vi "KM_Readout.vi"() -> ()   [LabVIEW 2015]
uses:
  <instrlib>/Zurich Instruments LabOne/Public/Data/ziTypePollType.ctl
  ZI_Frontpanel.ctl
  HF_FrontPanel.ctl
  <vilib>/Analysis/baseanly.llb/Mean (DBL).vi
  MQM Data Transfer_KM.vi
  <instrlib>/Zurich Instruments LabOne/Public/Data/ziGetEventAuxInSample.vi
  <instrlib>/Zurich Instruments LabOne/Public/Data/ziGetEventDemodSample.vi
  <instrlib>/Zurich Instruments LabOne/Zurich Instruments LabOne.lvlib
  <vilib>/Analysis/NI_AALBase.lvlib
panel:
  out "AUX Input 5":dbl[](graph)
  out "ziValueType 5":T1
  in  "stop 2":bool
  out "ZI HFLI":T2 {"Lockin 1 Demod 0"."R(V)" format="%#_6p"}
  out "ZI MFLI":T3 {"Lockin 1 Demod 3"."R(V)" format="%#_6p"; "Lockin 1 Demod 2"."R(V)" format="%#_6p"; "Lockin 4 Demod 1"."R(V)" format="%#_6p"; "Lockin 3 Demod 1"."R(V)" format="%#_6p"; "Lockin 2 Demod 1"."R(V)" format="%#_6p"; "Lockin 1 Demod 1"."R(V)" format="%#_6p"; "Lockin 4 Demod 0"."R(V)" format="%#_6p"; "Lockin 3 Demod 0"."R(V)" format="%#_6p"; "Lockin 2 Demod 0"."R(V)" format="%#_6p"; "Lockin 1 Demod 0"."R(V)" format="%#_6p"}
  out "AUX Input 4":dbl[](graph)
  out "ziValueType 4":T1
  out "AUX Input 3":dbl[](graph)
  out "ziValueType 3":T1
  out "AUX Input 2":dbl[](graph)
  out "ziValueType 2":T1
  in  "stop":bool
  out "ziValueType":T1
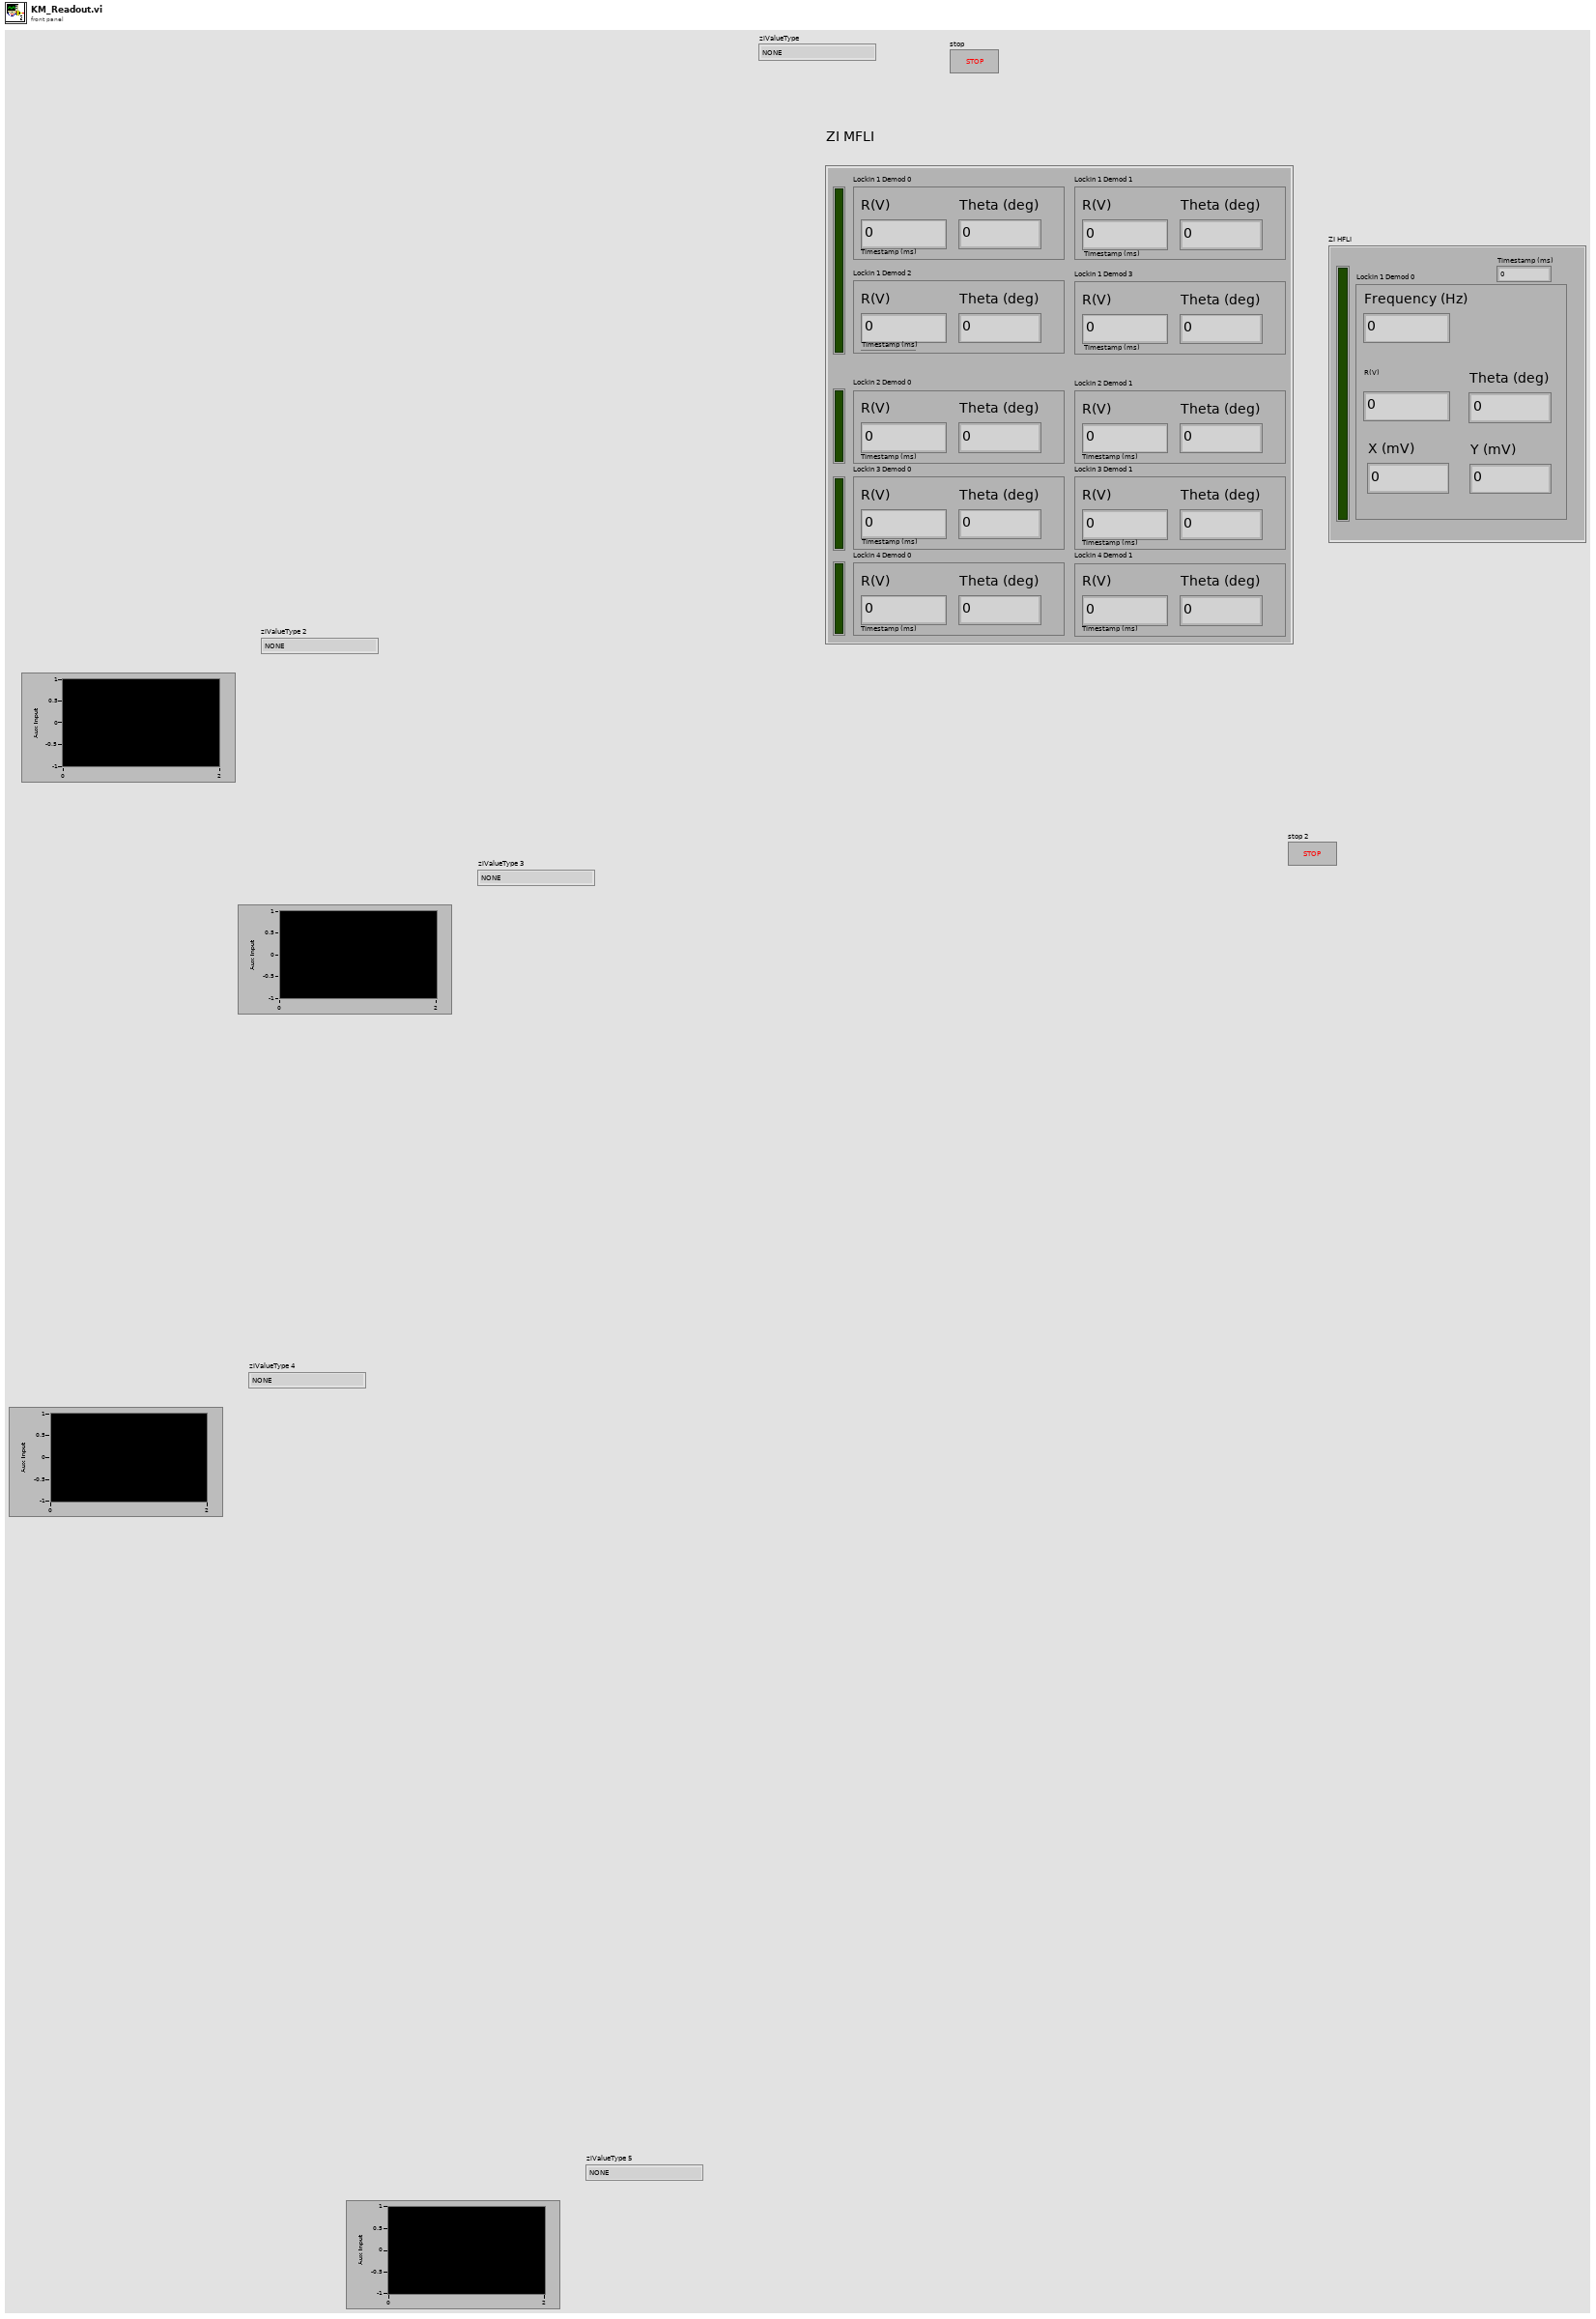
[diagram p1: front panel]
types:
  T1 = typedef "Zurich Instruments LabOne.lvlib/ziTypePollType.ctl" = enum16{"NONE", "DOUBLE_DATA", "INTEGER_DATA", "DEMOD_SAMPLE", "SCOPE_WAVE_HF2", "AUXIN_SAMPLE", "DIO_SAMPLE", "BYTE_ARRAY", "PWA_WAVE", "9", "10", "11", "12", "13", "14", "15", "TREE_CHANGE_DEPRI", "17", "ERROR", "19", "20", "21", "22", "23", "24", "25", "26", "27", "28", "29", "30", "31", "DOUBLE_DATA_TS", "INTEGER_DATA_TS", "34", "SCOPE_WAVE", "36", "37", "BYTE_ARRAY_TS", "39", "40", "41", "42", "43", "44", "45", "CNT_DATA", "47", "TREE_CHANGE", "49", "50", "51", "52", "53", "54", "55", "56", "57", "58", "59", "60", "61", "62", "63", "SWEEPER_DATA", "SPECTRUM_DATA", "ADVISOR_DATA", "67", "IMP_DATA"}
  T2 = typedef "HF_FrontPanel.ctl" = cluster{"Lockin 1 Demod 0":cluster{"R(V)":dbl, "Theta (deg)":dbl, "Frequency (Hz)":dbl, "X (mV)":dbl, "Y (mV)":dbl}, "LI1 active":bool, "Timestamp (ms)":u32}
  T3 = typedef "ZI_Frontpanel.ctl" = cluster{"Lockin 1 Demod 0":cluster{"R(V)":dbl, "Theta (deg)":dbl, "Timestamp (ms)":u32}, "Lockin 2 Demod 0":cluster{"R(V)":dbl, "Theta (deg)":dbl, "Timestamp (ms)":u32}, "Lockin 3 Demod 0":cluster{"R(V)":dbl, "Theta (deg)":dbl, "Timestamp (ms)":u32}, "Lockin 4 Demod 0":cluster{"R(V)":dbl, "Theta (deg)":dbl, "Timestamp (ms)":u32}, "Lockin 1 Demod 1":cluster{"R(V)":dbl, "Theta (deg)":dbl, "Timestamp (ms)":u32}, "Lockin 2 Demod 1":cluster{"R(V)":dbl, "Theta (deg)":dbl, "Timestamp (ms)":u32}, "Lockin 3 Demod 1":cluster{"R(V)":dbl, "Theta (deg)":dbl, "Timestamp (ms)":u32}, "Lockin 4 Demod 1":cluster{"R(V)":dbl, "Theta (deg)":dbl, "Timestamp (ms)":u32}, "Lockin 1 Demod 2":cluster{"R(V)":dbl, "Theta (deg)":dbl, "Timestamp (ms)":u32}, "Lockin 1 Demod 3":cluster{"R(V)":dbl, "Theta (deg)":dbl, "Timestamp (ms)":u32}, "LI1 active":bool, "LI2 active":bool, "LI3 active":bool, "LI4 active":bool}
  T4 = cluster{"ZI IP List[0]":string, "ZI IP List[1]":string, "ZI IP List[2]":string, "ZI IP List[3]":string, "ZI IP List[4]":string, "ZI IP List[5]":string, "ZI IP List[6]":string, "ZI IP List[7]":string, "ZI IP List[8]":string}
  T5 = typedef "Zurich Instruments LabOne.lvlib/ziTypeHandle.ctl" = cluster{"handleValid":bool, "Conn":u64, "Path Prefix":string, "Handle":u64, "Connected":bool, "Clockbase(s)":dbl}
  T6 = typedef "Zurich Instruments LabOne.lvlib/ziTypeAuxInSample.ctl" = cluster{"Timestamp (ticks)":u64[], "Val Ch0 (V)":dbl[], "Val Ch1 (V)":dbl[]}
  T7 = typedef "ziTypeDemodSampleEx.ctl" = cluster{"Timestamps (ticks)":u64[], "X (Vrms)":dbl[], "Y (Vrms)":dbl[], "Osc Phase (rad)":dbl[], "Freq (Hz)":dbl[], "DIO":u32[], "Aux In 0 (V)":dbl[], "Aux In 1 (V)":dbl[], "Trigger":u32[]}
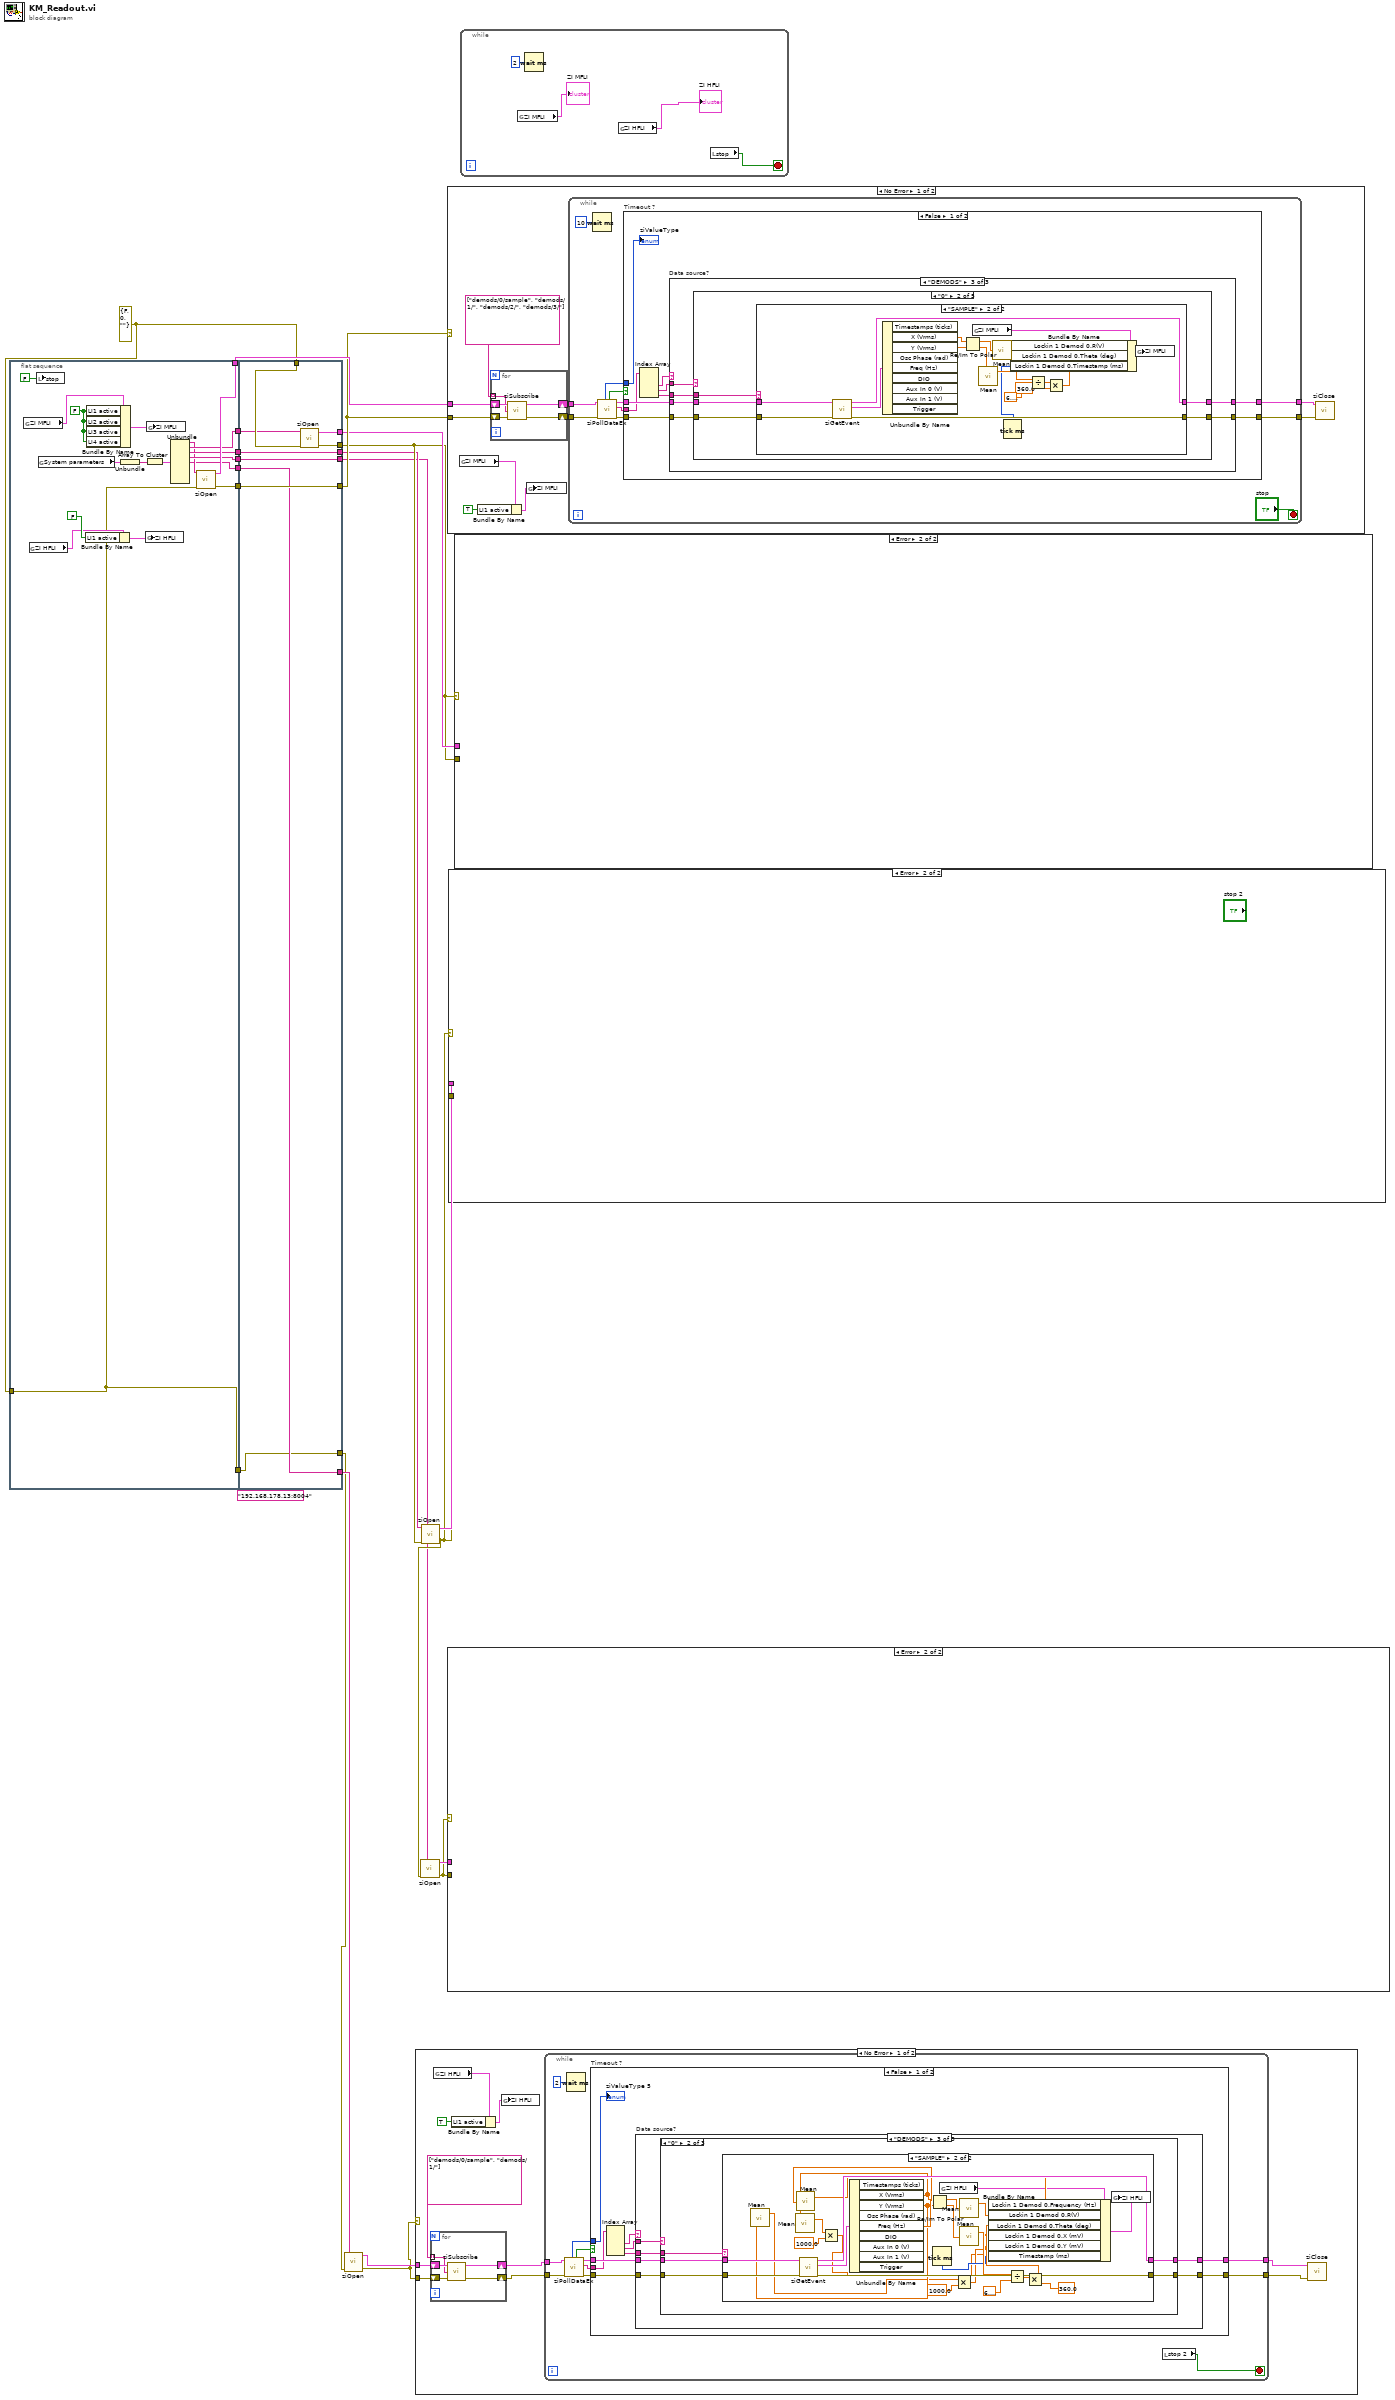
[diagram p0: block diagram]
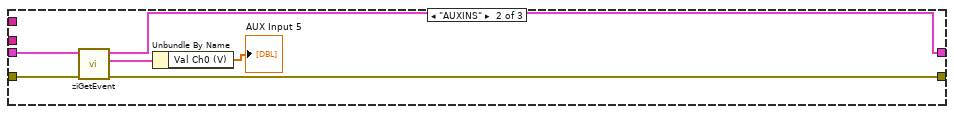
[diagram p3: hidden frame]
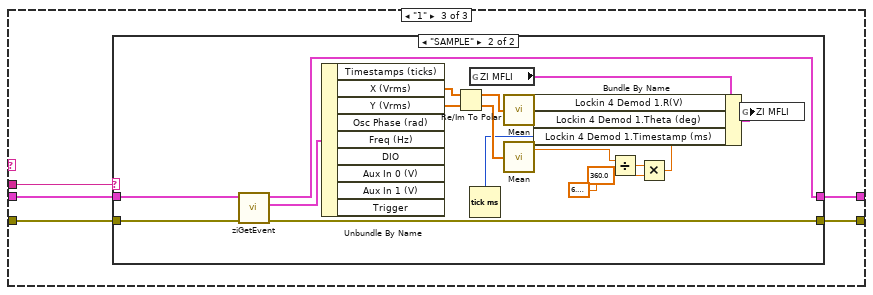
[diagram p6: hidden frame]
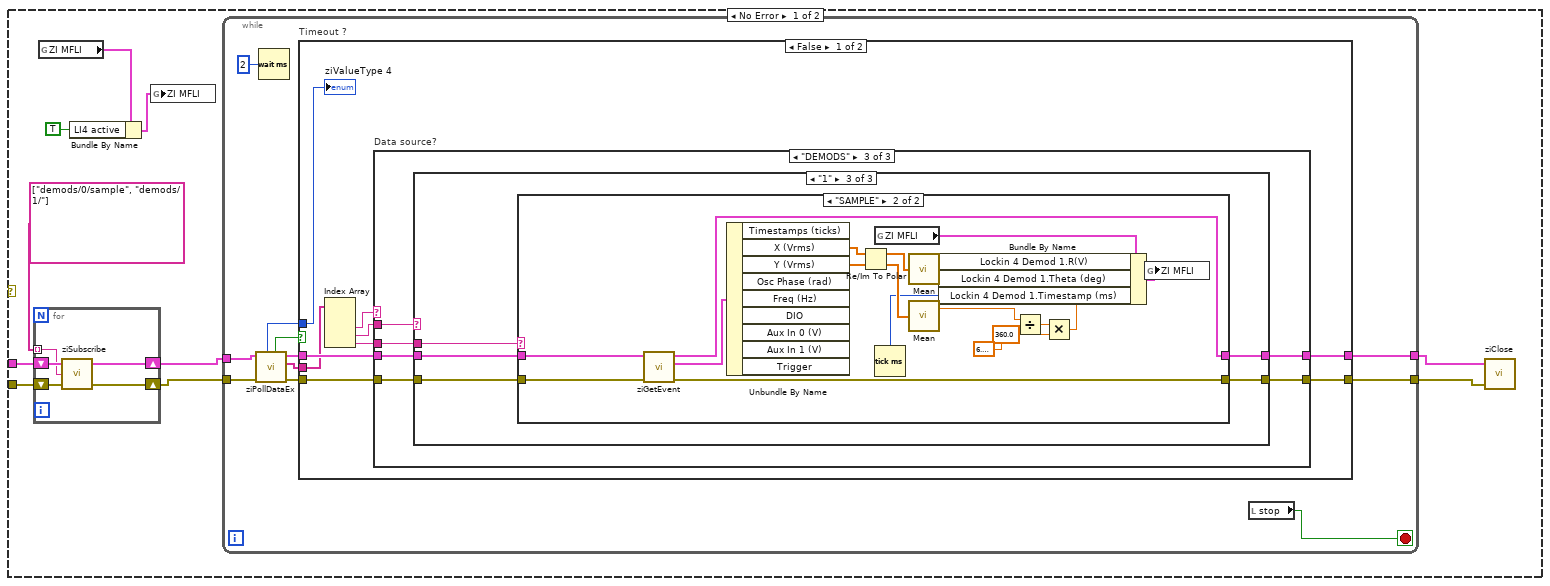
[diagram p10: hidden frame]
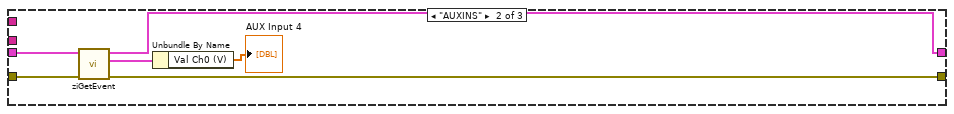
[diagram p12: hidden frame]
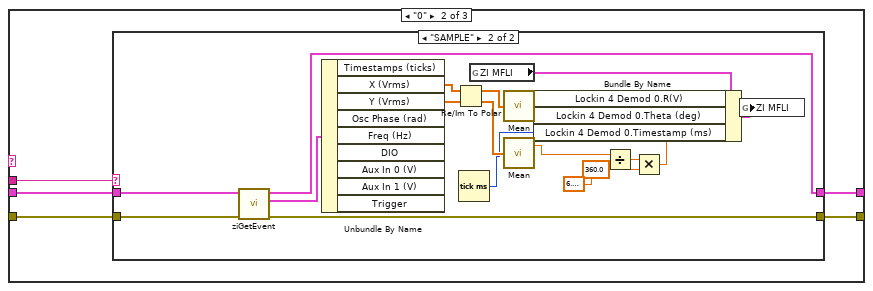
[diagram p14: hidden frame]
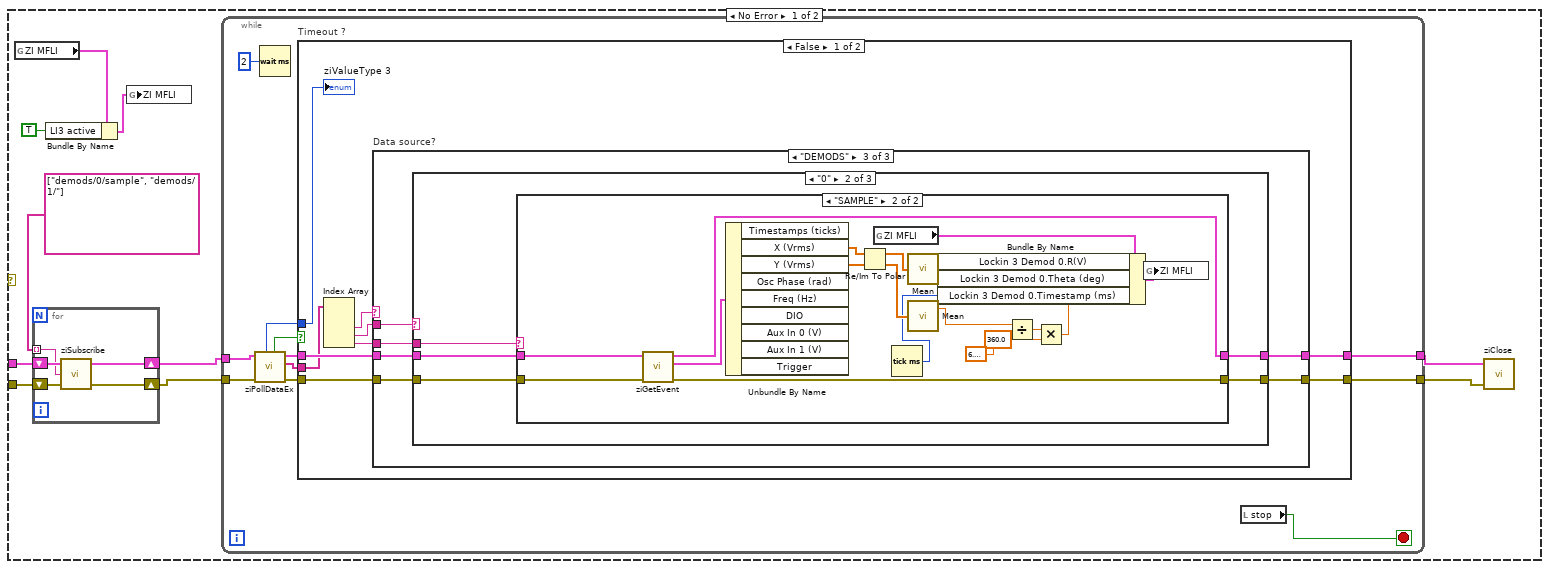
[diagram p18: hidden frame]
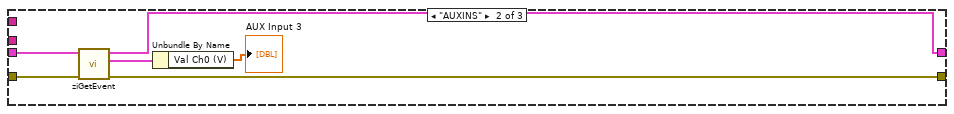
[diagram p20: hidden frame]
diagram:
  (unwired) "192.168.178.13:8004"
  w15 = errorcluster {"status"=FALSE, "code"=0, "source"=""} ("Error In")
  n1 = flat-sequence {
    tunnel: [w38] -> w19
    tunnel: [w37] -> w17
    tunnel: w15 -> [w22]
    tunnel: [w31] -> w12
    tunnel: [w30] -> w11
    tunnel: [w29] -> w10
    tunnel: [w23] -> w6
    tunnel: [w22] -> w2
    tunnel: [w48] -> w18
    tunnel: w17 -> [w48]
    tunnel: w15 -> [w47]
    tunnel: [w46] -> w14
    tunnel: [w45] -> w16
    tunnel: w12 -> [w44]
    tunnel: [w43] -> w9
    tunnel: w11 -> [w43]
    tunnel: [w42] -> w5
    tunnel: w10 -> [w42]
    tunnel: w6 -> [w41]
    tunnel: [w41] -> w4
    tunnel: w2 -> [w40]
    tunnel: [w40] -> w1
    frame #0 {
      w35 = FALSE ("LI1 active")
      n2 = global read "MQM Data Transfer_KM.vi" "ZI MFLI"() -> (w28:T3)
      n3 = global read "MQM Data Transfer_KM.vi" "ZI HFLI"() -> (w26:T2)
      n4 = local write "stop"(FALSE ("stop")) -> ()
      n5 = global read "MQM Data Transfer_KM.vi" "System parameters"() -> (w34:cluster{"ZI IP List":string[]})
      n6 = Bundle By Name(cluster=w26, "LI1 active"=FALSE) -> (w25:T2)
      n7 = Bundle By Name(cluster=w28, "LI1 active"=w35, "LI2 active"=w35, "LI3 active"=w35, "LI4 active"=w35) -> (w36:T3)
      n8 = Unbundle(w34) -> ("ZI IP List"=w33:string[])
      n9 = Array To Cluster(array=w33) -> (cluster=w32:T4)
      n10 = global write "MQM Data Transfer_KM.vi" "ZI HFLI"(w25) -> ()
      n11 = global write "MQM Data Transfer_KM.vi" "ZI MFLI"(w36) -> ()
      n12 = Unbundle(w32) -> ("ZI IP List[0]"=w24:string, "ZI IP List[1]"=w31:string, "ZI IP List[2]"=w30:string, "ZI IP List[3]"=w29:string, "ZI IP List[4]"=w23:string)  [unwired: 4 out]
      n13 = call <instrlib>:"ziOpen.vi"("Error In"=w22, "Address"=w24) -> ("Error Out"=w37:errorcluster, "HandleOut"=w38:T5)  [unwired: 3 out]
    }
    frame #1 {
      n14 = call <instrlib>:"ziOpen.vi"("Error In"=w47, "Address"=w44) -> ("Error Out"=w46:errorcluster, "HandleOut"=w45:T5)  [unwired: 3 out]
    }
  }
  n15 = call <instrlib>:"ziOpen.vi"("Error In"=w1, "Address"=w4) -> ("Error Out"=w7:errorcluster, "HandleOut"=w8:T5)  [unwired: 3 out]
  n16 = case shown="No Error" w7 {
    tunnel: w8 -> [w58 _]
    tunnel: w7 -> [w57 _]
    frame No Error {
      n17 = for {
        shift-right: [w63] -> w55
        shift-left: w58 -> [w61]
        shift-right: [w62] -> w54
        shift-left: w57 -> [w60]
        tunnel: string[] ["demods/0/sample", "demods/1/"] -> [w59] mode=indexing
        n18 = call <instrlib>:"ziSubscribe.vi"("error in"=w60, "Path ()"=w59, "Handle In"=w61) -> ("error out"=w62:errorcluster, "Handle Out"=w63:T5)  [unwired: 1 in]
      }
      n19 = global read "MQM Data Transfer_KM.vi" "ZI HFLI"() -> (w51:T2)
      n20 = Bundle By Name(cluster=w51, "LI1 active"=TRUE) -> (w49:T2)
      n21 = global write "MQM Data Transfer_KM.vi" "ZI HFLI"(w49) -> ()
      n22 = while {
        tunnel: w55 -> [w69]
        tunnel: w54 -> [w68]
        tunnel: [w67] -> w52
        tunnel: [w66] -> w53
        stop <- w65 stop-if-true
        n23 = call <instrlib>:"ziPollDataEx.vi"("error in"=w68, "Handle In"=w69) -> ("error out"=w72:errorcluster, "PathArray"=w70:string[], "Handle Out"=w74:T5, "Timed Out"=w73:bool, "ziValueType"=w71:T1)  [unwired: 2 in, 3 out]
        n24 = Wait (ms)(milliseconds to wait=u32 2) -> ()  [unwired: 1 out]
        n25 = case "Timeout ?" shown="False" w73 {
          tunnel: w74 -> [w83 w159]
          tunnel: [w82 w159] -> w66
          tunnel: w72 -> [w81 w158]
          tunnel: [w80 w158] -> w67
          tunnel: w71 -> [w79 _]
          tunnel: w70 -> [w78 _]
          frame False {
            n26 = Index Array(array=w78) -> (element #2=w75:string, element #3=w76:string, element #4=w77:string)  [unwired: 4 in, 1 out]
            n27 = case "Data source?" shown="\"DEMODS\"" w75 {
              tunnel: w83 -> [w85 w91 w97]
              tunnel: [w85 w89 w96] -> w82
              tunnel: w81 -> [w84 w88 w95]
              tunnel: [w84 w87 w94] -> w80
              tunnel: w76 -> [_ _ w93]
              tunnel: w77 -> [_ _ w92]
              frame Default {
              }
              frame "AUXINS" {
                n28 = call-poly <instrlib>:"ziGetEvent.vi"("Error In"=w88, "Handle In"=w91) -> ("Error Out"=w87:errorcluster, "AuxIn Out"=w90:T6, "Handle Out"=w89:T5)  [unwired: 7 in]
                n29 = Unbundle By Name(w90) -> ("Val Ch0 (V)"=→"AUX Input 5":dbl[])
              }
              frame "DEMODS" {
                n30 = case shown="\"0\"" w93 {
                  tunnel: w97 -> [w99 w104 w137]
                  tunnel: [w99 w103 w136] -> w96
                  tunnel: w95 -> [w98 w102 w135]
                  tunnel: [w98 w101 w134] -> w94
                  tunnel: w92 -> [_ w100 w133]
                  frame Default {
                  }
                  frame "0" {
                    n31 = case shown="\"SAMPLE\"" w100 {
                      tunnel: w104 -> [w106 w132]
                      tunnel: [w106 w130] -> w103
                      tunnel: w102 -> [w105 w129]
                      tunnel: [w105 w128] -> w101
                      frame Default {
                      }
                      frame "SAMPLE" {
                        n32 = call-poly <instrlib>:"ziGetEvent.vi"("Error In"=w129, "Handle In"=w132) -> ("Error Out"=w128:errorcluster, "Demod Sample Out"=w131:T7, "Handle Out"=w130:T5)  [unwired: 7 in]
                        n33 = Unbundle By Name(w131) -> ("X (Vrms)"=w116:dbl[], "Y (Vrms)"=w115:dbl[], "Freq (Hz)"=w118:dbl[])  [unwired: 6 out]
                        n34 = call-poly <vilib>:"Mean.vi"("X"=w115) -> ("mean"=w111:dbl)  [unwired: 1 out]
                        n35 = call-poly <vilib>:"Mean.vi"("X"=w116) -> ("mean"=w108:dbl)  [unwired: 1 out]
                        n36 = call-poly <vilib>:"Mean.vi"("X"=w118) -> ("mean"=w117:dbl)  [unwired: 1 out]
                        n37 = Multiply(x=w108, y=1000.0) -> (x*y=w107:dbl)
                        n38 = Re/Im To Polar(2:w115, 3:w116) -> (0:w126:dbl[], 1:w127:dbl[])
                        n39 = Tick Count (ms)() -> (millisecond timer value=w119:u32)
                        n40 = global read "MQM Data Transfer_KM.vi" "ZI HFLI"() -> (w114:T2)
                        n41 = Multiply(x=w111, y=1000.0) -> (x*y=w110:dbl)
                        n42 = call-poly <vilib>:"Mean.vi"("X"=w127) -> ("mean"=w122:dbl)  [unwired: 1 out]
                        n43 = call-poly <vilib>:"Mean.vi"("X"=w126) -> ("mean"=w121:dbl)  [unwired: 1 out]
                        n44 = Divide(x=w121, y=6.283185307179586) -> (x/y=w124:dbl)
                        n45 = Multiply(x=w124, y=360.0) -> (x*y=w120:dbl)
                        n46 = Bundle By Name(cluster=w114, "Lockin 1 Demod 0.Frequency (Hz)"=w117, "Lockin 1 Demod 0.R(V)"=w122, "Lockin 1 Demod 0.Theta (deg)"=w120, "Lockin 1 Demod 0.X (mV)"=w107, "Lockin 1 Demod 0.Y (mV)"=w110, "Timestamp (ms)"=w119) -> (w113:T2)
                        n47 = global write "MQM Data Transfer_KM.vi" "ZI HFLI"(w113) -> ()
                      }
                    }
                  }
                  frame "1" {
                    n48 = case shown="\"SAMPLE\"" w133 {
                      tunnel: w137 -> [w139 w155]
                      tunnel: [w139 w153] -> w136
                      tunnel: w135 -> [w138 w152]
                      tunnel: [w138 w151] -> w134
                      frame Default {
                      }
                      frame "SAMPLE" {
                        n49 = call-poly <instrlib>:"ziGetEvent.vi"("Error In"=w152, "Handle In"=w155) -> ("Error Out"=w151:errorcluster, "Demod Sample Out"=w154:T7, "Handle Out"=w153:T5)  [unwired: 7 in]
                        n50 = Unbundle By Name(w154) -> ("X (Vrms)"=w157:dbl[], "Y (Vrms)"=w156:dbl[])  [unwired: 7 out]
                        n51 = Re/Im To Polar(2:w156, 3:w157) -> (0:w149:dbl[], 1:w150:dbl[])
                        n52 = global read "MQM Data Transfer_KM.vi" "ZI MFLI"() -> (w148:T3)
                        n53 = Tick Count (ms)() -> (millisecond timer value=w140:u32)
                        n54 = call-poly <vilib>:"Mean.vi"("X"=w150) -> ("mean"=w146:dbl)  [unwired: 1 out]
                        n55 = call-poly <vilib>:"Mean.vi"("X"=w149) -> ("mean"=w142:dbl)  [unwired: 1 out]
                        n56 = Divide(x=w142, y=6.283185307179586) -> (x/y=w144:dbl)
                        n57 = Multiply(x=w144, y=360.0) -> (x*y=w141:dbl)
                        n58 = Bundle By Name(cluster=w148, "Lockin 4 Demod 1.R(V)"=w146, "Lockin 4 Demod 1.Theta (deg)"=w141, "Lockin 4 Demod 1.Timestamp (ms)"=w140) -> (w147:T3)
                        n59 = global write "MQM Data Transfer_KM.vi" "ZI MFLI"(w147) -> ()
                      }
                    }
                  }
                }
              }
            }
            "ziValueType 5" <- w79
          }
          frame True {
            # "Timeout, no action."
          }
        }
        n60 = local read "stop 2"() -> (w65:bool)
      }
      n61 = call "ziClose.vi"("Error In"=w52, "Handle In"=w53) -> ()  [unwired: 4 out]
    }
    frame Error {
    }
  }
  n62 = call <instrlib>:"ziOpen.vi"("Error In"=w14, "Address"=w9) -> ("Error Out"=w13:errorcluster, "HandleOut"=w21:T5)  [unwired: 3 out]
  n63 = call <instrlib>:"ziOpen.vi"("Error In"=w13, "Address"=w5) -> ("Error Out"=w3:errorcluster, "HandleOut"=w20:T5)  [unwired: 3 out]
  n64 = case shown="Error" w3 {
    tunnel: w20 -> [w169 _]
    tunnel: w3 -> [w168 _]
    frame No Error {
      n65 = for {
        shift-right: [w174] -> w166
        shift-left: w169 -> [w172]
        shift-right: [w173] -> w165
        shift-left: w168 -> [w171]
        tunnel: string[] ["demods/0/sample", "demods/1/"] -> [w170] mode=indexing
        n66 = call <instrlib>:"ziSubscribe.vi"("error in"=w171, "Path ()"=w170, "Handle In"=w172) -> ("error out"=w173:errorcluster, "Handle Out"=w174:T5)  [unwired: 1 in]
      }
      n67 = global read "MQM Data Transfer_KM.vi" "ZI MFLI"() -> (w162:T3)
      n68 = Bundle By Name(cluster=w162, "LI4 active"=TRUE ("LI1 active")) -> (w160:T3)
      n69 = global write "MQM Data Transfer_KM.vi" "ZI MFLI"(w160) -> ()
      n70 = while {
        tunnel: w166 -> [w180]
        tunnel: w165 -> [w179]
        tunnel: [w178] -> w163
        tunnel: [w177] -> w164
        stop <- w176 stop-if-true
        n71 = call <instrlib>:"ziPollDataEx.vi"("error in"=w179, "Handle In"=w180) -> ("error out"=w183:errorcluster, "PathArray"=w181:string[], "Handle Out"=w185:T5, "Timed Out"=w184:bool, "ziValueType"=w182:T1)  [unwired: 2 in, 3 out]
        n72 = Wait (ms)(milliseconds to wait=u32 2) -> ()  [unwired: 1 out]
        n73 = case "Timeout ?" shown="False" w184 {
          tunnel: w185 -> [w194 w262]
          tunnel: [w193 w262] -> w177
          tunnel: w183 -> [w192 w261]
          tunnel: [w191 w261] -> w178
          tunnel: w182 -> [w190 _]
          tunnel: w181 -> [w189 _]
          frame False {
            n74 = Index Array(array=w189) -> (element #2=w186:string, element #3=w187:string, element #4=w188:string)  [unwired: 4 in, 1 out]
            n75 = case "Data source?" shown="\"DEMODS\"" w186 {
              tunnel: w194 -> [w196 w202 w208]
              tunnel: [w196 w200 w207] -> w193
              tunnel: w192 -> [w195 w199 w206]
              tunnel: [w195 w198 w205] -> w191
              tunnel: w187 -> [_ _ w204]
              tunnel: w188 -> [_ _ w203]
              frame Default {
              }
              frame "AUXINS" {
                n76 = call-poly <instrlib>:"ziGetEvent.vi"("Error In"=w199, "Handle In"=w202) -> ("Error Out"=w198:errorcluster, "AuxIn Out"=w201:T6, "Handle Out"=w200:T5)  [unwired: 7 in]
                n77 = Unbundle By Name(w201) -> ("Val Ch0 (V)"=→"AUX Input 4":dbl[])
              }
              frame "DEMODS" {
                n78 = case shown="\"1\"" w204 {
                  tunnel: w208 -> [w210 w215 w240]
                  tunnel: [w210 w214 w239] -> w207
                  tunnel: w206 -> [w209 w213 w238]
                  tunnel: [w209 w212 w237] -> w205
                  tunnel: w203 -> [_ w211 w236]
                  frame Default {
                  }
                  frame "0" {
                    n79 = case shown="\"SAMPLE\"" w211 {
                      tunnel: w215 -> [w217 w233]
                      tunnel: [w217 w231] -> w214
                      tunnel: w213 -> [w216 w230]
                      tunnel: [w216 w229] -> w212
                      frame Default {
                      }
                      frame "SAMPLE" {
                        n80 = call-poly <instrlib>:"ziGetEvent.vi"("Error In"=w230, "Handle In"=w233) -> ("Error Out"=w229:errorcluster, "Demod Sample Out"=w232:T7, "Handle Out"=w231:T5)  [unwired: 7 in]
                        n81 = Unbundle By Name(w232) -> ("X (Vrms)"=w235:dbl[], "Y (Vrms)"=w234:dbl[])  [unwired: 7 out]
                        n82 = Re/Im To Polar(2:w234, 3:w235) -> (0:w224:dbl[], 1:w225:dbl[])
                        n83 = Tick Count (ms)() -> (millisecond timer value=w218:u32)
                        n84 = global read "MQM Data Transfer_KM.vi" "ZI MFLI"() -> (w228:T3)
                        n85 = call-poly <vilib>:"Mean.vi"("X"=w225) -> ("mean"=w226:dbl)  [unwired: 1 out]
                        n86 = call-poly <vilib>:"Mean.vi"("X"=w224) -> ("mean"=w220:dbl)  [unwired: 1 out]
                        n87 = Divide(x=w220, y=6.283185307179586) -> (x/y=w222:dbl)
                        n88 = Multiply(x=w222, y=360.0) -> (x*y=w219:dbl)
                        n89 = Bundle By Name(cluster=w228, "Lockin 4 Demod 0.R(V)"=w226, "Lockin 4 Demod 0.Theta (deg)"=w219, "Lockin 4 Demod 0.Timestamp (ms)"=w218) -> (w227:T3)
                        n90 = global write "MQM Data Transfer_KM.vi" "ZI MFLI"(w227) -> ()
                      }
                    }
                  }
                  frame "1" {
                    n91 = case shown="\"SAMPLE\"" w236 {
                      tunnel: w240 -> [w242 w258]
                      tunnel: [w242 w256] -> w239
                      tunnel: w238 -> [w241 w255]
                      tunnel: [w241 w254] -> w237
                      frame Default {
                      }
                      frame "SAMPLE" {
                        n92 = call-poly <instrlib>:"ziGetEvent.vi"("Error In"=w255, "Handle In"=w258) -> ("Error Out"=w254:errorcluster, "Demod Sample Out"=w257:T7, "Handle Out"=w256:T5)  [unwired: 7 in]
                        n93 = Unbundle By Name(w257) -> ("X (Vrms)"=w260:dbl[], "Y (Vrms)"=w259:dbl[])  [unwired: 7 out]
                        n94 = Re/Im To Polar(2:w259, 3:w260) -> (0:w252:dbl[], 1:w253:dbl[])
                        n95 = global read "MQM Data Transfer_KM.vi" "ZI MFLI"() -> (w251:T3)
                        n96 = Tick Count (ms)() -> (millisecond timer value=w243:u32)
                        n97 = call-poly <vilib>:"Mean.vi"("X"=w253) -> ("mean"=w249:dbl)  [unwired: 1 out]
                        n98 = call-poly <vilib>:"Mean.vi"("X"=w252) -> ("mean"=w245:dbl)  [unwired: 1 out]
                        n99 = Divide(x=w245, y=6.283185307179586) -> (x/y=w247:dbl)
                        n100 = Multiply(x=w247, y=360.0) -> (x*y=w244:dbl)
                        n101 = Bundle By Name(cluster=w251, "Lockin 4 Demod 1.R(V)"=w249, "Lockin 4 Demod 1.Theta (deg)"=w244, "Lockin 4 Demod 1.Timestamp (ms)"=w243) -> (w250:T3)
                        n102 = global write "MQM Data Transfer_KM.vi" "ZI MFLI"(w250) -> ()
                      }
                    }
                  }
                }
              }
            }
            "ziValueType 4" <- w190
          }
          frame True {
            # "Timeout, no action."
          }
        }
        n103 = local read "stop"() -> (w176:bool)
      }
      n104 = call "ziClose.vi"("Error In"=w163, "Handle In"=w164) -> ()  [unwired: 4 out]
    }
    frame Error {
    }
  }
  n105 = case shown="No Error" w18 {
    tunnel: w19 -> [w272 _]
    tunnel: w18 -> [w266 _]
    frame No Error {
      n106 = global read "MQM Data Transfer_KM.vi" "ZI MFLI"() -> (w265:T3)
      n107 = Bundle By Name(cluster=w265, "LI1 active"=TRUE) -> (w263:T3)
      n108 = for {
        shift-right: [w414] -> w271
        shift-left: w272 -> [w412]
        shift-right: [w413] -> w270
        shift-left: w266 -> [w411]
        tunnel: string[] ["demods/0/sample", "demods/1/", "demods/2/", "demods/3/"] -> [w410] mode=indexing
        n109 = call <instrlib>:"ziSubscribe.vi"("error in"=w411, "Path ()"=w410, "Handle In"=w412) -> ("error out"=w413:errorcluster, "Handle Out"=w414:T5)  [unwired: 1 in]
      }
      n110 = global write "MQM Data Transfer_KM.vi" "ZI MFLI"(w263) -> ()
      n111 = while {
        tunnel: w271 -> [w278]
        tunnel: w270 -> [w277]
        tunnel: [w276] -> w268
        tunnel: [w275] -> w267
        stop <- "stop" stop-if-true
        n112 = Wait (ms)(milliseconds to wait=u32 10) -> ()  [unwired: 1 out]
        n113 = call <instrlib>:"ziPollDataEx.vi"("error in"=w277, "Handle In"=w278) -> ("error out"=w281:errorcluster, "PathArray"=w279:string[], "Handle Out"=w283:T5, "Timed Out"=w282:bool, "ziValueType"=w280:T1)  [unwired: 2 in, 3 out]
        n114 = case "Timeout ?" shown="False" w282 {
          tunnel: w283 -> [w292 w409]
          tunnel: [w291 w409] -> w275
          tunnel: w281 -> [w290 w408]
          tunnel: [w289 w408] -> w276
          tunnel: w280 -> [w288 _]
          tunnel: w279 -> [w287 _]
          frame False {
            n115 = Index Array(array=w287) -> (element #2=w284:string, element #3=w285:string, element #4=w286:string)  [unwired: 4 in, 1 out]
            n116 = case "Data source?" shown="\"DEMODS\"" w284 {
              tunnel: w292 -> [w294 w299 w305]
              tunnel: [w294 w297 w304] -> w291
              tunnel: w290 -> [w293 w296 w303]
              tunnel: [w293 w295 w302] -> w289
              tunnel: w285 -> [_ _ w301]
              tunnel: w286 -> [_ _ w300]
              frame Default {
              }
              frame "AUXINS" {
                n117 = call-poly <instrlib>:"ziGetEvent.vi"("Error In"=w296, "Handle In"=w299) -> ("Error Out"=w295:errorcluster, "AuxIn Out"=w298:T6, "Handle Out"=w297:T5)  [unwired: 7 in]
                n118 = Unbundle By Name(w298) -> ()  [unwired: 1 out]
              }
              frame "DEMODS" {
                n119 = case shown="\"0\"" w301 {
                  tunnel: w305 -> [w307 w312 w337 w362 w387]
                  tunnel: [w307 w311 w336 w361 w386] -> w304
                  tunnel: w303 -> [w306 w310 w335 w360 w385]
                  tunnel: [w306 w309 w334 w359 w384] -> w302
                  tunnel: w300 -> [_ w308 w333 w358 w383]
                  frame Default {
                  }
                  frame "0" {
                    n120 = case shown="\"SAMPLE\"" w308 {
                      tunnel: w312 -> [w314 w330]
                      tunnel: [w314 w328] -> w311
                      tunnel: w310 -> [w313 w327]
                      tunnel: [w313 w326] -> w309
                      frame Default {
                      }
                      frame "SAMPLE" {
                        n121 = call-poly <instrlib>:"ziGetEvent.vi"("Error In"=w327, "Handle In"=w330) -> ("Error Out"=w326:errorcluster, "Demod Sample Out"=w329:T7, "Handle Out"=w328:T5)  [unwired: 7 in]
                        n122 = Unbundle By Name(w329) -> ("X (Vrms)"=w332:dbl[], "Y (Vrms)"=w331:dbl[])  [unwired: 7 out]
                        n123 = Re/Im To Polar(2:w331, 3:w332) -> (0:w321:dbl[], 1:w322:dbl[])
                        n124 = global read "MQM Data Transfer_KM.vi" "ZI MFLI"() -> (w325:T3)
                        n125 = call-poly <vilib>:"Mean.vi"("X"=w321) -> ("mean"=w320:dbl)  [unwired: 1 out]
                        n126 = call-poly <vilib>:"Mean.vi"("X"=w322) -> ("mean"=w323:dbl)  [unwired: 1 out]
                        n127 = Tick Count (ms)() -> (millisecond timer value=w315:u32)
                        n128 = Divide(x=w320, y=6.283185307179586) -> (x/y=w318:dbl)
                        n129 = Multiply(x=w318, y=360.0) -> (x*y=w316:dbl)
                        n130 = Bundle By Name(cluster=w325, "Lockin 1 Demod 0.R(V)"=w323, "Lockin 1 Demod 0.Theta (deg)"=w316, "Lockin 1 Demod 0.Timestamp (ms)"=w315) -> (w324:T3)
                        n131 = global write "MQM Data Transfer_KM.vi" "ZI MFLI"(w324) -> ()
                      }
                    }
                  }
                  frame "1" {
                    n132 = case shown="\"SAMPLE\"" w333 {
                      tunnel: w337 -> [w339 w355]
                      tunnel: [w339 w353] -> w336
                      tunnel: w335 -> [w338 w352]
                      tunnel: [w338 w351] -> w334
                      frame Default {
                      }
                      frame "SAMPLE" {
                        n133 = call-poly <instrlib>:"ziGetEvent.vi"("Error In"=w352, "Handle In"=w355) -> ("Error Out"=w351:errorcluster, "Demod Sample Out"=w354:T7, "Handle Out"=w353:T5)  [unwired: 7 in]
                        n134 = Unbundle By Name(w354) -> ("X (Vrms)"=w357:dbl[], "Y (Vrms)"=w356:dbl[])  [unwired: 7 out]
                        n135 = Re/Im To Polar(2:w356, 3:w357) -> (0:w349:dbl[], 1:w350:dbl[])
                        n136 = global read "MQM Data Transfer_KM.vi" "ZI MFLI"() -> (w348:T3)
                        n137 = Tick Count (ms)() -> (millisecond timer value=w340:u32)
                        n138 = call-poly <vilib>:"Mean.vi"("X"=w350) -> ("mean"=w346:dbl)  [unwired: 1 out]
                        n139 = call-poly <vilib>:"Mean.vi"("X"=w349) -> ("mean"=w342:dbl)  [unwired: 1 out]
                        n140 = Divide(x=w342, y=6.283185307179586) -> (x/y=w344:dbl)
                        n141 = Multiply(x=w344, y=360.0) -> (x*y=w341:dbl)
                        n142 = Bundle By Name(cluster=w348, "Lockin 1 Demod 1.R(V)"=w346, "Lockin 1 Demod 1.Theta (deg)"=w341, "Lockin 1 Demod 1.Timestamp (ms)"=w340) -> (w347:T3)
                        n143 = global write "MQM Data Transfer_KM.vi" "ZI MFLI"(w347) -> ()
                      }
                    }
                  }
                  frame "2" {
                    n144 = case shown="\"SAMPLE\"" w358 {
                      tunnel: w362 -> [w364 w380]
                      tunnel: [w364 w378] -> w361
                      tunnel: w360 -> [w363 w377]
                      tunnel: [w363 w376] -> w359
                      frame Default {
                      }
                      frame "SAMPLE" {
                        n145 = call-poly <instrlib>:"ziGetEvent.vi"("Error In"=w377, "Handle In"=w380) -> ("Error Out"=w376:errorcluster, "Demod Sample Out"=w379:T7, "Handle Out"=w378:T5)  [unwired: 7 in]
                        n146 = Unbundle By Name(w379) -> ("X (Vrms)"=w382:dbl[], "Y (Vrms)"=w381:dbl[])  [unwired: 7 out]
                        n147 = Tick Count (ms)() -> (millisecond timer value=w365:u32)
                        n148 = Re/Im To Polar(2:w381, 3:w382) -> (0:w374:dbl[], 1:w375:dbl[])
                        n149 = global read "MQM Data Transfer_KM.vi" "ZI MFLI"() -> (w373:T3)
                        n150 = call-poly <vilib>:"Mean.vi"("X"=w375) -> ("mean"=w371:dbl)  [unwired: 1 out]
                        n151 = call-poly <vilib>:"Mean.vi"("X"=w374) -> ("mean"=w367:dbl)  [unwired: 1 out]
                        n152 = Divide(x=w367, y=6.283185307179586) -> (x/y=w369:dbl)
                        n153 = Multiply(x=w369, y=360.0) -> (x*y=w366:dbl)
                        n154 = Bundle By Name(cluster=w373, "Lockin 1 Demod 2.R(V)"=w371, "Lockin 1 Demod 2.Theta (deg)"=w366, "Lockin 1 Demod 2.Timestamp (ms)"=w365) -> (w372:T3)
                        n155 = global write "MQM Data Transfer_KM.vi" "ZI MFLI"(w372) -> ()
                      }
                    }
                  }
                  frame "3" {
                    n156 = case shown="\"SAMPLE\"" w383 {
                      tunnel: w387 -> [w389 w405]
                      tunnel: [w389 w403] -> w386
                      tunnel: w385 -> [w388 w402]
                      tunnel: [w388 w401] -> w384
                      frame Default {
                      }
                      frame "SAMPLE" {
                        n157 = call-poly <instrlib>:"ziGetEvent.vi"("Error In"=w402, "Handle In"=w405) -> ("Error Out"=w401:errorcluster, "Demod Sample Out"=w404:T7, "Handle Out"=w403:T5)  [unwired: 7 in]
                        n158 = Unbundle By Name(w404) -> ("X (Vrms)"=w407:dbl[], "Y (Vrms)"=w406:dbl[])  [unwired: 7 out]
                        n159 = Re/Im To Polar(2:w406, 3:w407) -> (0:w399:dbl[], 1:w400:dbl[])
                        n160 = global read "MQM Data Transfer_KM.vi" "ZI MFLI"() -> (w398:T3)
                        n161 = Tick Count (ms)() -> (millisecond timer value=w390:u32)
                        n162 = call-poly <vilib>:"Mean.vi"("X"=w400) -> ("mean"=w396:dbl)  [unwired: 1 out]
                        n163 = call-poly <vilib>:"Mean.vi"("X"=w399) -> ("mean"=w392:dbl)  [unwired: 1 out]
                        n164 = Divide(x=w392, y=6.283185307179586) -> (x/y=w394:dbl)
                        n165 = Multiply(x=w394, y=360.0) -> (x*y=w391:dbl)
                        n166 = Bundle By Name(cluster=w398, "Lockin 1 Demod 3.R(V)"=w396, "Lockin 1 Demod 3.Theta (deg)"=w391, "Lockin 1 Demod 3.Timestamp (ms)"=w390) -> (w397:T3)
                        n167 = global write "MQM Data Transfer_KM.vi" "ZI MFLI"(w397) -> ()
                      }
                    }
                  }
                }
              }
            }
            "ziValueType" <- w288
          }
          frame True {
            # "Timeout, no action."
          }
        }
      }
      n168 = call "ziClose.vi"("Error In"=w268, "Handle In"=w267) -> ()  [unwired: 4 out]
    }
    frame Error {
    }
  }
  n169 = case shown="Error" w13 {
    tunnel: w21 -> [w424 _]
    tunnel: w13 -> [w423 _]
    frame No Error {
      n170 = global read "MQM Data Transfer_KM.vi" "ZI MFLI"() -> (w417:T3)
      n171 = for {
        shift-right: [w429] -> w421
        shift-left: w424 -> [w427]
        shift-right: [w428] -> w420
        shift-left: w423 -> [w426]
        tunnel: string[] ["demods/0/sample", "demods/1/"] -> [w425] mode=indexing
        n172 = call <instrlib>:"ziSubscribe.vi"("error in"=w426, "Path ()"=w425, "Handle In"=w427) -> ("error out"=w428:errorcluster, "Handle Out"=w429:T5)  [unwired: 1 in]
      }
      n173 = Bundle By Name(cluster=w417, "LI3 active"=TRUE ("LI1 active")) -> (w415:T3)
      n174 = global write "MQM Data Transfer_KM.vi" "ZI MFLI"(w415) -> ()
      n175 = while {
        tunnel: w421 -> [w435]
        tunnel: w420 -> [w434]
        tunnel: [w433] -> w418
        tunnel: [w432] -> w419
        stop <- w431 stop-if-true
        n176 = call <instrlib>:"ziPollDataEx.vi"("error in"=w434, "Handle In"=w435) -> ("error out"=w438:errorcluster, "PathArray"=w436:string[], "Handle Out"=w440:T5, "Timed Out"=w439:bool, "ziValueType"=w437:T1)  [unwired: 2 in, 3 out]
        n177 = Wait (ms)(milliseconds to wait=u32 2) -> ()  [unwired: 1 out]
        n178 = case "Timeout ?" shown="False" w439 {
          tunnel: w440 -> [w449 w517]
          tunnel: [w448 w517] -> w432
          tunnel: w438 -> [w447 w516]
          tunnel: [w446 w516] -> w433
          tunnel: w437 -> [w445 _]
          tunnel: w436 -> [w444 _]
          frame False {
            n179 = Index Array(array=w444) -> (element #2=w441:string, element #3=w442:string, element #4=w443:string)  [unwired: 4 in, 1 out]
            n180 = case "Data source?" shown="\"DEMODS\"" w441 {
              tunnel: w449 -> [w451 w457 w463]
              tunnel: [w451 w455 w462] -> w448
              tunnel: w447 -> [w450 w454 w461]
              tunnel: [w450 w453 w460] -> w446
              tunnel: w442 -> [_ _ w459]
              tunnel: w443 -> [_ _ w458]
              frame Default {
              }
              frame "AUXINS" {
                n181 = call-poly <instrlib>:"ziGetEvent.vi"("Error In"=w454, "Handle In"=w457) -> ("Error Out"=w453:errorcluster, "AuxIn Out"=w456:T6, "Handle Out"=w455:T5)  [unwired: 7 in]
                n182 = Unbundle By Name(w456) -> ("Val Ch0 (V)"=→"AUX Input 3":dbl[])
              }
              frame "DEMODS" {
                n183 = case shown="\"0\"" w459 {
                  tunnel: w463 -> [w465 w470 w495]
                  tunnel: [w465 w469 w494] -> w462
                  tunnel: w461 -> [w464 w468 w493]
                  tunnel: [w464 w467 w492] -> w460
                  tunnel: w458 -> [_ w466 w491]
                  frame Default {
                  }
                  frame "0" {
                    n184 = case shown="\"SAMPLE\"" w466 {
                      tunnel: w470 -> [w472 w488]
                      tunnel: [w472 w486] -> w469
                      tunnel: w468 -> [w471 w485]
                      tunnel: [w471 w484] -> w467
                      frame Default {
                      }
                      frame "SAMPLE" {
                        n185 = call-poly <instrlib>:"ziGetEvent.vi"("Error In"=w485, "Handle In"=w488) -> ("Error Out"=w484:errorcluster, "Demod Sample Out"=w487:T7, "Handle Out"=w486:T5)  [unwired: 7 in]
                        n186 = Unbundle By Name(w487) -> ("X (Vrms)"=w490:dbl[], "Y (Vrms)"=w489:dbl[])  [unwired: 7 out]
                        n187 = Re/Im To Polar(2:w489, 3:w490) -> (0:w479:dbl[], 1:w480:dbl[])
                        n188 = global read "MQM Data Transfer_KM.vi" "ZI MFLI"() -> (w483:T3)
                        n189 = Tick Count (ms)() -> (millisecond timer value=w473:u32)
                        n190 = call-poly <vilib>:"Mean.vi"("X"=w480) -> ("mean"=w481:dbl)  [unwired: 1 out]
                        n191 = call-poly <vilib>:"Mean.vi"("X"=w479) -> ("mean"=w475:dbl)  [unwired: 1 out]
                        n192 = Divide(x=w475, y=6.283185307179586) -> (x/y=w477:dbl)
                        n193 = Multiply(x=w477, y=360.0) -> (x*y=w474:dbl)
                        n194 = Bundle By Name(cluster=w483, "Lockin 3 Demod 0.R(V)"=w481, "Lockin 3 Demod 0.Theta (deg)"=w474, "Lockin 3 Demod 0.Timestamp (ms)"=w473) -> (w482:T3)
                        n195 = global write "MQM Data Transfer_KM.vi" "ZI MFLI"(w482) -> ()
                      }
                    }
                  }
                  frame "1" {
                    n196 = case shown="\"SAMPLE\"" w491 {
                      tunnel: w495 -> [w497 w513]
                      tunnel: [w497 w511] -> w494
                      tunnel: w493 -> [w496 w510]
                      tunnel: [w496 w509] -> w492
                      frame Default {
                      }
                      frame "SAMPLE" {
                        n197 = call-poly <instrlib>:"ziGetEvent.vi"("Error In"=w510, "Handle In"=w513) -> ("Error Out"=w509:errorcluster, "Demod Sample Out"=w512:T7, "Handle Out"=w511:T5)  [unwired: 7 in]
                        n198 = Unbundle By Name(w512) -> ("X (Vrms)"=w515:dbl[], "Y (Vrms)"=w514:dbl[])  [unwired: 7 out]
                        n199 = Re/Im To Polar(2:w514, 3:w515) -> (0:w507:dbl[], 1:w508:dbl[])
                        n200 = global read "MQM Data Transfer_KM.vi" "ZI MFLI"() -> (w506:T3)
                        n201 = Tick Count (ms)() -> (millisecond timer value=w498:u32)
                        n202 = call-poly <vilib>:"Mean.vi"("X"=w508) -> ("mean"=w504:dbl)  [unwired: 1 out]
                        n203 = call-poly <vilib>:"Mean.vi"("X"=w507) -> ("mean"=w500:dbl)  [unwired: 1 out]
                        n204 = Divide(x=w500, y=6.283185307179586) -> (x/y=w502:dbl)
                        n205 = Multiply(x=w502, y=360.0) -> (x*y=w499:dbl)
                        n206 = Bundle By Name(cluster=w506, "Lockin 3 Demod 1.R(V)"=w504, "Lockin 3 Demod 1.Theta (deg)"=w499, "Lockin 3 Demod 1.Timestamp (ms)"=w498) -> (w505:T3)
                        n207 = global write "MQM Data Transfer_KM.vi" "ZI MFLI"(w505) -> ()
                      }
                    }
                  }
                }
              }
            }
            "ziValueType 3" <- w445
          }
          frame True {
            # "Timeout, no action."
          }
        }
        n208 = local read "stop"() -> (w431:bool)
      }
      n209 = call "ziClose.vi"("Error In"=w418, "Handle In"=w419) -> ()  [unwired: 4 out]
    }
    frame Error {
    }
  }
  n210 = case shown="Error" w14 {
    tunnel: w16 -> [w527 _]
    tunnel: w14 -> [w526 _]
    frame No Error {
      n211 = global read "MQM Data Transfer_KM.vi" "ZI MFLI"() -> (w520:T3)
      n212 = Bundle By Name(cluster=w520, "LI2 active"=TRUE ("LI1 active")) -> (w518:T3)
      n213 = for {
        shift-right: [w532] -> w525
        shift-left: w527 -> [w530]
        shift-right: [w531] -> w524
        shift-left: w526 -> [w529]
        tunnel: string[] ["demods/0/sample", "demods/1/"] -> [w528] mode=indexing
        n214 = call <instrlib>:"ziSubscribe.vi"("error in"=w529, "Path ()"=w528, "Handle In"=w530) -> ("error out"=w531:errorcluster, "Handle Out"=w532:T5)  [unwired: 1 in]
      }
      n215 = global write "MQM Data Transfer_KM.vi" "ZI MFLI"(w518) -> ()
      n216 = while {
        tunnel: w525 -> [w538]
        tunnel: w524 -> [w537]
        tunnel: [w536] -> w522
        tunnel: [w535] -> w521
        stop <- w534 stop-if-true
        n217 = call <instrlib>:"ziPollDataEx.vi"("error in"=w537, "Handle In"=w538) -> ("error out"=w541:errorcluster, "PathArray"=w539:string[], "Handle Out"=w543:T5, "Timed Out"=w542:bool, "ziValueType"=w540:T1)  [unwired: 2 in, 3 out]
        n218 = Wait (ms)(milliseconds to wait=u32 2) -> ()  [unwired: 1 out]
        n219 = case "Timeout ?" shown="False" w542 {
          tunnel: w543 -> [w552 w620]
          tunnel: [w551 w620] -> w535
          tunnel: w541 -> [w550 w619]
          tunnel: [w549 w619] -> w536
          tunnel: w540 -> [w548 _]
          tunnel: w539 -> [w547 _]
          frame False {
            n220 = Index Array(array=w547) -> (element #2=w544:string, element #3=w545:string, element #4=w546:string)  [unwired: 4 in, 1 out]
            n221 = case "Data source?" shown="\"DEMODS\"" w544 {
              tunnel: w552 -> [w554 w560 w566]
              tunnel: [w554 w558 w565] -> w551
              tunnel: w550 -> [w553 w557 w564]
              tunnel: [w553 w556 w563] -> w549
              tunnel: w545 -> [_ _ w562]
              tunnel: w546 -> [_ _ w561]
              frame Default {
              }
              frame "AUXINS" {
                n222 = call-poly <instrlib>:"ziGetEvent.vi"("Error In"=w557, "Handle In"=w560) -> ("Error Out"=w556:errorcluster, "AuxIn Out"=w559:T6, "Handle Out"=w558:T5)  [unwired: 7 in]
                n223 = Unbundle By Name(w559) -> ("Val Ch0 (V)"=→"AUX Input 2":dbl[])
              }
              frame "DEMODS" {
                n224 = case shown="\"1\"" w562 {
                  tunnel: w566 -> [w568 w573 w598]
                  tunnel: [w568 w572 w597] -> w565
                  tunnel: w564 -> [w567 w571 w596]
                  tunnel: [w567 w570 w595] -> w563
                  tunnel: w561 -> [_ w569 w594]
                  frame Default {
                  }
                  frame "0" {
                    n225 = case shown="\"SAMPLE\"" w569 {
                      tunnel: w573 -> [w575 w591]
                      tunnel: [w575 w589] -> w572
                      tunnel: w571 -> [w574 w588]
                      tunnel: [w574 w587] -> w570
                      frame Default {
                      }
                      frame "SAMPLE" {
                        n226 = call-poly <instrlib>:"ziGetEvent.vi"("Error In"=w588, "Handle In"=w591) -> ("Error Out"=w587:errorcluster, "Demod Sample Out"=w590:T7, "Handle Out"=w589:T5)  [unwired: 7 in]
                        n227 = Unbundle By Name(w590) -> ("X (Vrms)"=w593:dbl[], "Y (Vrms)"=w592:dbl[])  [unwired: 7 out]
                        n228 = Re/Im To Polar(2:w592, 3:w593) -> (0:w582:dbl[], 1:w583:dbl[])
                        n229 = global read "MQM Data Transfer_KM.vi" "ZI MFLI"() -> (w586:T3)
                        n230 = Tick Count (ms)() -> (millisecond timer value=w576:u32)
                        n231 = call-poly <vilib>:"Mean.vi"("X"=w583) -> ("mean"=w584:dbl)  [unwired: 1 out]
                        n232 = call-poly <vilib>:"Mean.vi"("X"=w582) -> ("mean"=w578:dbl)  [unwired: 1 out]
                        n233 = Divide(x=w578, y=6.283185307179586) -> (x/y=w580:dbl)
                        n234 = Multiply(x=w580, y=360.0) -> (x*y=w577:dbl)
                        n235 = Bundle By Name(cluster=w586, "Lockin 2 Demod 0.R(V)"=w584, "Lockin 2 Demod 0.Theta (deg)"=w577, "Lockin 2 Demod 0.Timestamp (ms)"=w576) -> (w585:T3)
                        n236 = global write "MQM Data Transfer_KM.vi" "ZI MFLI"(w585) -> ()
                      }
                    }
                  }
                  frame "1" {
                    n237 = case shown="\"SAMPLE\"" w594 {
                      tunnel: w598 -> [w600 w616]
                      tunnel: [w600 w614] -> w597
                      tunnel: w596 -> [w599 w613]
                      tunnel: [w599 w612] -> w595
                      frame Default {
                      }
                      frame "SAMPLE" {
                        n238 = call-poly <instrlib>:"ziGetEvent.vi"("Error In"=w613, "Handle In"=w616) -> ("Error Out"=w612:errorcluster, "Demod Sample Out"=w615:T7, "Handle Out"=w614:T5)  [unwired: 7 in]
                        n239 = Unbundle By Name(w615) -> ("X (Vrms)"=w618:dbl[], "Y (Vrms)"=w617:dbl[])  [unwired: 7 out]
                        n240 = Re/Im To Polar(2:w617, 3:w618) -> (0:w610:dbl[], 1:w611:dbl[])
                        n241 = global read "MQM Data Transfer_KM.vi" "ZI MFLI"() -> (w609:T3)
                        n242 = Tick Count (ms)() -> (millisecond timer value=w601:u32)
                        n243 = call-poly <vilib>:"Mean.vi"("X"=w611) -> ("mean"=w607:dbl)  [unwired: 1 out]
                        n244 = call-poly <vilib>:"Mean.vi"("X"=w610) -> ("mean"=w603:dbl)  [unwired: 1 out]
                        n245 = Divide(x=w603, y=6.283185307179586) -> (x/y=w605:dbl)
                        n246 = Multiply(x=w605, y=360.0) -> (x*y=w602:dbl)
                        n247 = Bundle By Name(cluster=w609, "Lockin 2 Demod 1.R(V)"=w607, "Lockin 2 Demod 1.Theta (deg)"=w602, "Lockin 2 Demod 1.Timestamp (ms)"=w601) -> (w608:T3)
                        n248 = global write "MQM Data Transfer_KM.vi" "ZI MFLI"(w608) -> ()
                      }
                    }
                  }
                }
              }
            }
            "ziValueType 2" <- w548
          }
          frame True {
            # "Timeout, no action."
          }
        }
        n249 = local read "stop"() -> (w534:bool)
      }
      n250 = call "ziClose.vi"("Error In"=w522, "Handle In"=w521) -> ()  [unwired: 4 out]
    }
    frame Error {
    }
  }
  n251 = while {
    stop <- w623 stop-if-true
    n252 = global read "MQM Data Transfer_KM.vi" "ZI MFLI"() -> (→"ZI MFLI":T3)
    n253 = Wait (ms)(milliseconds to wait=u32 2) -> ()  [unwired: 1 out]
    n254 = global read "MQM Data Transfer_KM.vi" "ZI HFLI"() -> (→"ZI HFLI":T2)
    n255 = local read "stop"() -> (w623:bool)
  }
